vi "SaveBallNOLPFData.vi"() -> ()   [LabVIEW 2017]
uses:
  <vilib>/Utility/file.llb/Write To Spreadsheet File (DBL).vi
panel:
  in  "file path (dialog if empty)":path
  in  "stop":bool
  in  "Sampling rate(Hz)":dbl=50.0
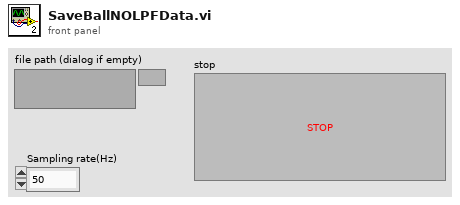
[diagram p1: front panel]
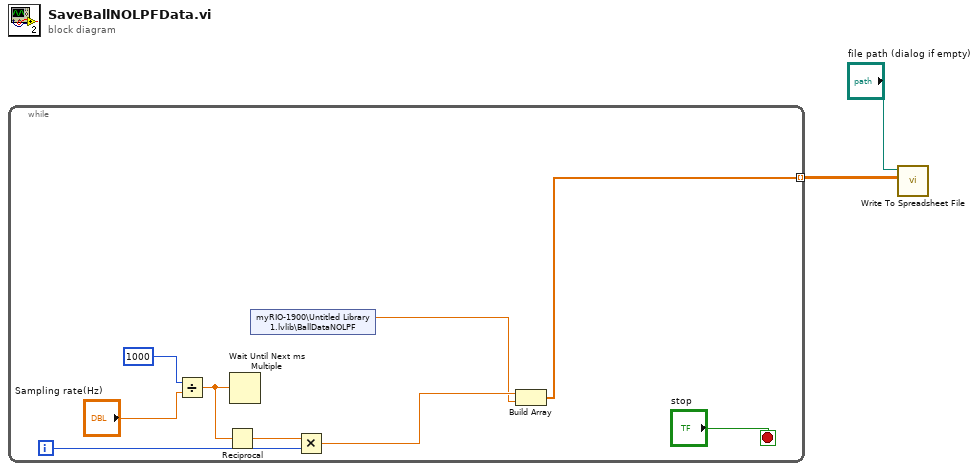
[diagram p0: block diagram]
diagram:
  n1 = while {
    tunnel: [w4] -> w1 mode=indexing
    i -> [w5]
    stop <- "stop" stop-if-true
    n2 = Divide(x=1000, y="Sampling rate(Hz)") -> (x/y=w7:dbl)
    n3 = Reciprocal(x=w7) -> (1/x=w6:dbl)
    n4 = Wait Until Next ms Multiple(millisecond multiple=w7) -> ()  [unwired: 1 out]
    n5 = shared-variable "myRIO-1900\\Untitled Library 1.lvlib\\BallDataNOLPF"() -> (w3:dbl)  [unwired: 1 in, 1 out]
    n6 = Multiply(x=w6, y=w5) -> (x*y=w10:dbl)
    n7 = Build Array(w10, w3) -> (w4:dbl[])
  }
  n8 = call-poly <vilib>:"Write To Spreadsheet File.vi"("2D data"=w1, "file path (dialog if empty)"="file path (dialog if empty)") -> ()  [unwired: 6 in, 1 out]
